vi "Init selected Camera.vi"(8 "error in":errorcluster, 11 "IMG_SRC in":refnum<class "IMG_SRC.lvclass">) -> (0 "error out":errorcluster, 3 "IMG_SRC out":refnum<class "IMG_SRC.lvclass">)   [LabVIEW 2018, in "IMG_SRC.lvlib" / "IMG_SRC.lvclass"]
uses:
  IMG_SRC.lvclass
  IMG_SRC.lvclass/IMG_SRC.ctl
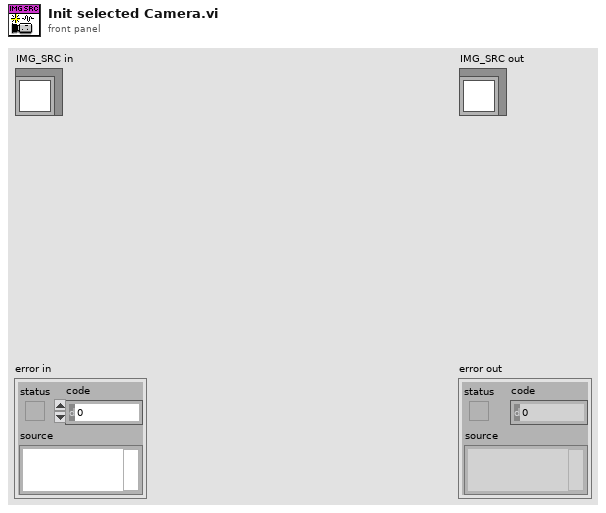
[diagram p1: front panel]
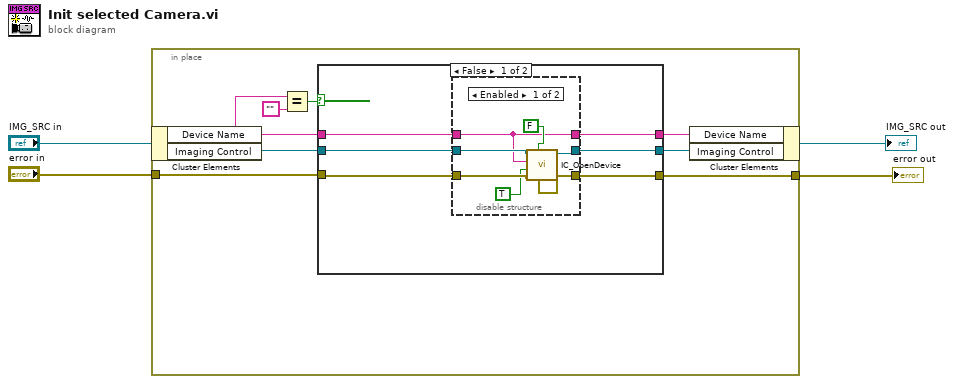
[diagram p0: block diagram]
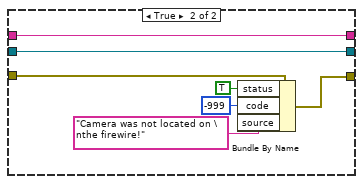
[diagram p3: hidden frame]
diagram:
  n1 = in-place {
    in-place-border: "error in" -> [w8]
    in-place-border: [w5] -> w1
    n2 = in-place-cluster #1("IMG_SRC in") -> ("Device Name"=w9:string, "Imaging Control"=w10:refnum<k7>)
    n3 = Equal?(x=w9, y="") -> (x = y?=w11:bool)
    n4 = case shown="False" w11 {
      tunnel: w8 -> [w15 w30]
      tunnel: [w18 w32] -> w6
      tunnel: w9 -> [w17 w31]
      tunnel: w10 -> [w14 w32]
      tunnel: [w13 w31] -> w7
      tunnel: [w16 w29] -> w5
      frame False {
        n5 = disable-structure shown="Enabled" {
          disable-tunnel: [w24 w28] -> w18
          disable-tunnel: w17 -> [w19 w26]
          disable-tunnel: [w22 w27] -> w16
          disable-tunnel: w15 -> [w23 w27]
          disable-tunnel: w14 -> [w25 w28]
          disable-tunnel: [w19 w26] -> w13
          frame Enabled {
            n6 = call <userlib>:"IC_OpenDevice.vi"("Color"=FALSE, "Error In (no error)"=w23, "Live"=TRUE, "Device"=w19, "ICImagingControl In"=w25) -> ("ICImagingControl Out"=w24:refnum<k7>, "Error Out"=w22:errorcluster)  [unwired: 1 in, 4 out]
          }
          frame Disabled {
          }
        }
      }
      frame True {
        n7 = Bundle By Name(cluster=w30, "status"=TRUE, "code"=-999, "source"="Camera was not located on \nthe firewire!") -> (w29:errorcluster)
      }
    }
    n8 = in-place-cluster #1("Device Name"=w7, "Imaging Control"=w6) -> (→"IMG_SRC out":refnum<class "IMG_SRC.lvclass">)
  }
  "error out" <- w1
